vi "make_mt_wf.vi"(9 "dt":dbl=1.0, 10 "t0":dbl, 11 "Y":cdb[](array[numeric])) -> (3 "output MT waveform":cluster{"t0":dbl, "dt":dbl, "Y":cdb[]})   [LabVIEW 2012]
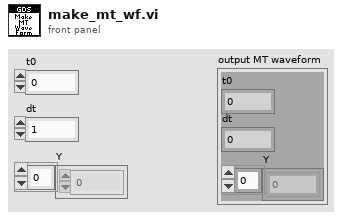
[diagram p1: front panel]
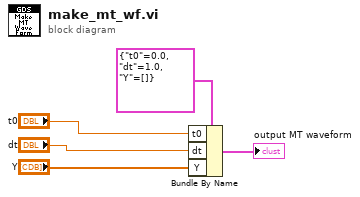
[diagram p0: block diagram]
diagram:
  n1 = Bundle By Name(cluster=cluster{"t0":dbl, "dt":dbl, "Y":cdb[]} {"t0"=0.0, "dt"=1.0, "Y"=[]} ("IQ data (complex) in"), "t0"="t0", "dt"="dt", "Y"="Y") -> (→"output MT waveform":cluster{"t0":dbl, "dt":dbl, "Y":cdb[]})
